vi "Global 1_diag.vi"() -> ()   [LabVIEW 2015]
panel:
  out "Measurement File":path
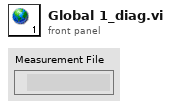
[diagram p1: front panel]
diagram:
